vi "tsdb_get_lin_db_frame_properties_by_db_index.vi"(8 "error in (no error)":errorcluster caption="错误输入（无错误）", 9 "AIndex":i32, 10 "AIdxDB":i32, 11 "路径输入":path=path "D:/Program Files (x86)/TOSUN/TSMaster/bin/TSMaster.dll") -> (0 "error out":errorcluster caption="错误输出", 1 "TDBFrameProperties":T1, 2 "function return":i32, 3 "路径输出":path)   [LabVIEW 2014]
doc: "Function Introduction\nRetrieve frame attributes of a specified LIN database through database index\nCall location\ninput parameter \nAIdxDB: Database Index\nAIndes: Index\nAvalue: The returned attribute data structure, please search for the definition in the TSMaster header\nReturn value\n==0: Execution successful\nOther values: Query error code"
uses:
  Typedef/TDBFrameProperties.ctl
panel:
  # "// TDBFrameProperties for database Frame properties, size = 1088\ntypedef struct _TDBFrameProperties {\n    s32 FDBIndex;\n    s32 FECUIndex;\n    s32 FFrameIndex;\n    u8  FIsTx;    \n    u8  FReserved1;\n    u16 FCycleTimeMs;\n    TSignalType FFrameType;\n    // CAN\n    u8  FCANIsDataFrame;\n    u8  FCANIsStdFrame;\n    u8  FCANIsEdl;\n    u8  FCANIsBrs;\n    s32 FCANIdentifier;\n    s32 FCANDLC;\n    s32 FCANDataBytes;\n    // LIN\n    s32 FLINIdentifier;\n    s32 FLINDLC;\n    // FlexRay\n    u8  FFRChannelMask;\n    u8  FFRBaseCycle;\n    u8  FFRCycleRepetition;\n    u8  FFRIsStartupFrame;\n    u16 FFRSlotId;  \n    u16 FFRDLC;\n    u64 FFRCycleMask;\n    s32 FSignalCount;\n    char FName[DATABASE_STR_LEN];\n    char FComment[DATABASE_STR_LEN];\n} TDBFrameProperties, *PDBFrameProperties;"
  # "// TDBFrameProperties for database Frame properties, size = 1088\ntypedef struct _TDBFrameProperties {\n    s32 FDBIndex;\n    s32 FECUIndex;\n    s32 FFrameIndex;\n    u8  FIsTx;    \n    u8  FReserved1;\n    u16 FCycleTimeMs;\n    TSignalType FFrameType;\n    // CAN\n    u8  FCANIsDataFrame;\n    u8  FCANIsStdFrame;\n    u8  FCANIsEdl;\n    u8  FCANIsBrs;\n    s32 FCANIdentifier;\n    s32 FCANDLC;\n    s32 FCANDataBytes;\n    // LIN\n    s32 FLINIdentifier;\n    s32 FLINDLC;\n    // FlexRay\n    u8  FFRChannelMask;\n    u8  FFRBaseCycle;\n    u8  FFRCycleRepetition;\n    u8  FFRIsStartupFrame;\n    u16 FFRSlotId;  \n    u16 FFRDLC;\n    u64 FFRCycleMask;\n    s32 FSignalCount;\n    char FName[DATABASE_STR_LEN];\n    char FComment[DATABASE_STR_LEN];\n} TDBFrameProperties, *PDBFrameProperties;"
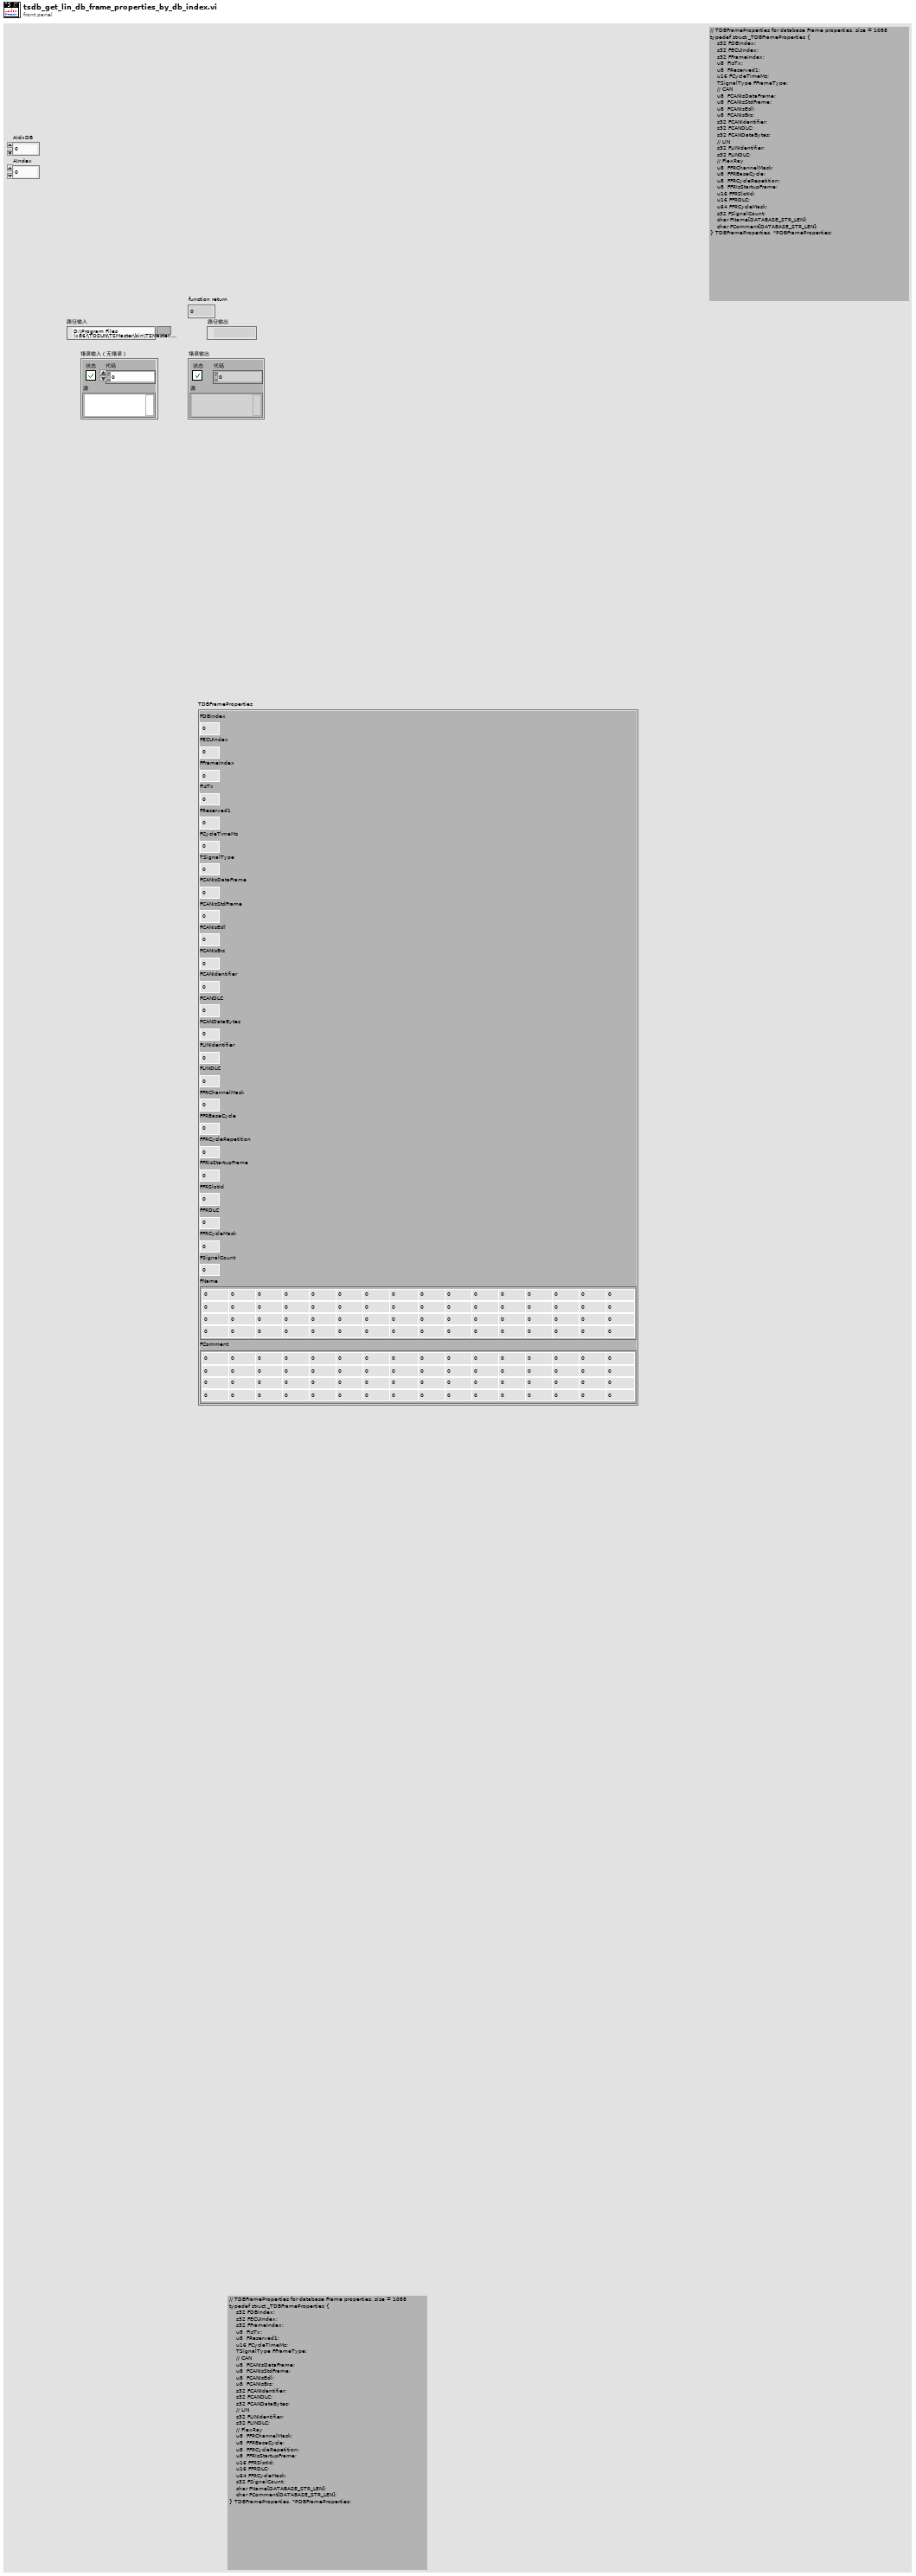
[diagram p1: front panel]
types:
  T1 = typedef "TDBFrameProperties.ctl" = cluster{"FDBIndex":i32, "FECUIndex":i32, "FFrameIndex":i32, "FIsTx":u8, "FReserved1":u8, "FCycleTimeMs":u16, "TSignalType":i32, "FCANIsDataFrame":u8, "FCANIsStdFrame":u8, "FCANIsEdl":u8, "FCANIsBrs":u8, "FCANIdentifier":i32, "FCANDLC":i32, "FCANDataBytes":i32, "FLINIdentifier":i32, "FLINDLC":i32, "FFRChannelMask":u8, "FFRBaseCycle":u8, "FFRCycleRepetition":u8, "FFRIsStartupFrame":u8, "FFRSlotId":u16, "FFRDLC":u16, "FFRCycleMask":u64, "FSignalCount":i32, "FName":cluster{"数值":u64, "数值 2":u64, "数值 3":u64, "数值 4":u64, "数值 5":u64, "数值 6":u64, "数值 7":u64, "数值 8":u64, "数值 9":u64, "数值 10":u64, "数值 11":u64, "数值 12":u64, "数值 13":u64, "数值 14":u64, "数值 15":u64, "数值 16":u64, "数值 17":u64, "数值 18":u64, "数值 19":u64, "数值 20":u64, "数值 21":u64, "数值 22":u64, "数值 23":u64, "数值 24":u64, "数值 25":u64, "数值 26":u64, "数值 27":u64, "数值 28":u64, "数值 29":u64, "数值 30":u64, "数值 31":u64, "数值 32":u64, "数值 33":u64, "数值 34":u64, "数值 35":u64, "数值 36":u64, "数值 37":u64, "数值 38":u64, "数值 39":u64, "数值 40":u64, "数值 41":u64, "数值 42":u64, "数值 43":u64, "数值 44":u64, "数值 45":u64, "数值 46":u64, "数值 47":u64, "数值 48":u64, "数值 49":u64, "数值 50":u64, "数值 51":u64, "数值 52":u64, "数值 53":u64, "数值 54":u64, "数值 55":u64, "数值 56":u64, "数值 57":u64, "数值 58":u64, "数值 59":u64, "数值 60":u64, "数值 61":u64, "数值 62":u64, "数值 63":u64, "数值 64":u64}, "FComment":cluster{"数值":u64, "数值 2":u64, "数值 3":u64, "数值 4":u64, "数值 5":u64, "数值 6":u64, "数值 7":u64, "数值 8":u64, "数值 9":u64, "数值 10":u64, "数值 11":u64, "数值 12":u64, "数值 13":u64, "数值 14":u64, "数值 15":u64, "数值 16":u64, "数值 17":u64, "数值 18":u64, "数值 19":u64, "数值 20":u64, "数值 21":u64, "数值 22":u64, "数值 23":u64, "数值 24":u64, "数值 25":u64, "数值 26":u64, "数值 27":u64, "数值 28":u64, "数值 29":u64, "数值 30":u64, "数值 31":u64, "数值 32":u64, "数值 33":u64, "数值 34":u64, "数值 35":u64, "数值 36":u64, "数值 37":u64, "数值 38":u64, "数值 39":u64, "数值 40":u64, "数值 41":u64, "数值 42":u64, "数值 43":u64, "数值 44":u64, "数值 45":u64, "数值 46":u64, "数值 47":u64, "数值 48":u64, "数值 49":u64, "数值 50":u64, "数值 51":u64, "数值 52":u64, "数值 53":u64, "数值 54":u64, "数值 55":u64, "数值 56":u64, "数值 57":u64, "数值 58":u64, "数值 59":u64, "数值 60":u64, "数值 61":u64, "数值 62":u64, "数值 63":u64, "数值 64":u64}}
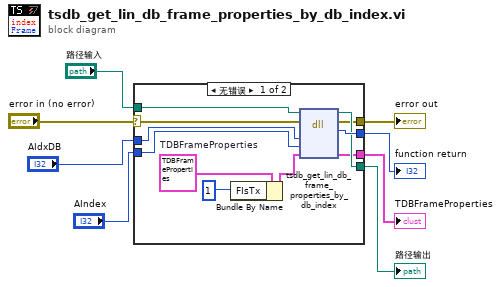
[diagram p0: block diagram]
diagram:
  n1 = case shown="无错误" "error in (no error)" {
    selector: "error in (no error)" -> [w13 w20]
    tunnel: [w19 _] -> w8
    tunnel: "路径输入" -> [w18 w21]
    tunnel: [w17 w21] -> w6
    tunnel: [w16 w20] -> w5
    tunnel: [w15 _] -> w4
    tunnel: "AIdxDB" -> [w14 _]
    tunnel: "AIndex" -> [w11 _]
    frame No Error {
      w12 = T1 {"FDBIndex"=0, "FECUIndex"=0, "FFrameIndex"=0, "FIsTx"=0, "FReserved1"=0, "FCycleTimeMs"=0, "TSignalType"=0, "FCANIsDataFrame"=0, "FCANIsStdFrame"=0, "FCANIsEdl"=0, "FCANIsBrs"=0, "FCANIdentifier"=0, "FCANDLC"=0, "FCANDataBytes"=0, "FLINIdentifier"=0, "FLINDLC"=0, "FFRChannelMask"=0, "FFRBaseCycle"=0, "FFRCycleRepetition"=0, "FFRIsStartupFrame"=0, "FFRSlotId"=0, "FFRDLC"=0, "FFRCycleMask"=0, "FSignalCount"=0, "FName"={"数值"=0, "数值 2"=0, "数值 3"=0, "数值 4"=0, "数值 5"=0, "数值 6"=0, "数值 7"=0, "数值 8"=0, "数值 9"=0, "数值 10"=0, "数值 11"=0, "数值 12"=0, "数值 13"=0, "数值 14"=0, "数值 15"=0, "数值 16"=0, "数值 17"=0, "数值 18"=0, "数值 19"=0, "数值 20"=0, "数值 21"=0, "数值 22"=0, "数值 23"=0, "数值 24"=0, "数值 25"=0, "数值 26"=0, "数值 27"=0, "数值 28"=0, "数值 29"=0, "数值 30"=0, "数值 31"=0, "数值 32"=0, "数值 33"=0, "数值 34"=0, "数值 35"=0, "数值 36"=0, "数值 37"=0, "数值 38"=0, "数值 39"=0, "数值 40"=0, "数值 41"=0, "数值 42"=0, "数值 43"=0, "数值 44"=0, "数值 45"=0, "数值 46"=0, "数值 47"=0, "数值 48"=0, "数值 49"=0, "数值 50"=0, "数值 51"=0, "数值 52"=0, "数值 53"=0, "数值 54"=0, "数值 55"=0, "数值 56"=0, "数值 57"=0, "数值 58"=0, "数值 59"=0, "数值 60"=0, "数值 61"=0, "数值 62"=0, "数值 63"=0, "数值 64"=0}, "FComment"={"数值"=0, "数值 2"=0, "数值 3"=0, "数值 4"=0, "数值 5"=0, "数值 6"=0, "数值 7"=0, "数值 8"=0, "数值 9"=0, "数值 10"=0, "数值 11"=0, "数值 12"=0, "数值 13"=0, "数值 14"=0, "数值 15"=0, "数值 16"=0, "数值 17"=0, "数值 18"=0, "数值 19"=0, "数值 20"=0, "数值 21"=0, "数值 22"=0, "数值 23"=0, "数值 24"=0, "数值 25"=0, "数值 26"=0, "数值 27"=0, "数值 28"=0, "数值 29"=0, "数值 30"=0, "数值 31"=0, "数值 32"=0, "数值 33"=0, "数值 34"=0, "数值 35"=0, "数值 36"=0, "数值 37"=0, "数值 38"=0, "数值 39"=0, "数值 40"=0, "数值 41"=0, "数值 42"=0, "数值 43"=0, "数值 44"=0, "数值 45"=0, "数值 46"=0, "数值 47"=0, "数值 48"=0, "数值 49"=0, "数值 50"=0, "数值 51"=0, "数值 52"=0, "数值 53"=0, "数值 54"=0, "数值 55"=0, "数值 56"=0, "数值 57"=0, "数值 58"=0, "数值 59"=0, "数值 60"=0, "数值 61"=0, "数值 62"=0, "数值 63"=0, "数值 64"=0}}  # TDBFrameProperties
      n2 = Bundle By Name(cluster=w12, "FIsTx"=u8 1) -> (w10:T1)
      n3 = dll-call lib="D:/Work/LabVIEW Code/TSMaster Labview SDK/LabVIEW/LabVIEW-TSMasterAPI_CLN/TSMasterAPI_LabVIEW-2024-08-27 16-32-25/Not_organized_vi/TSMaster.*" fn="tsdb_get_lin_db_frame_properties_by_db_index"(path in=w18, error in=w13, "AIdxDB"=w14, "AIndex"=w11, "Avalue"=w10) -> (path out=w17:path, error out=w16:errorcluster, "返回类型"=w19:i32, "Avalue"=w15:T1)  [unwired: 3 in]
    }
    frame Error {
    }
  }
  "function return" <- w8
  "error out" <- w5
  "路径输出" <- w6
  "TDBFrameProperties" <- w4
